vi "Write Post Office Addresses.vi"(8 "error in (no error)":errorcluster, 10 "Post Office Addresses":string[](array[string]), 11 "Post in":refnum<class "Post.lvclass">) -> (0 "error out":errorcluster, 3 "Post out":refnum<class "Post.lvclass">)   [LabVIEW 2019, in "Post.lvclass"]
uses:
  Post.lvclass
  Post.lvclass/Post.ctl
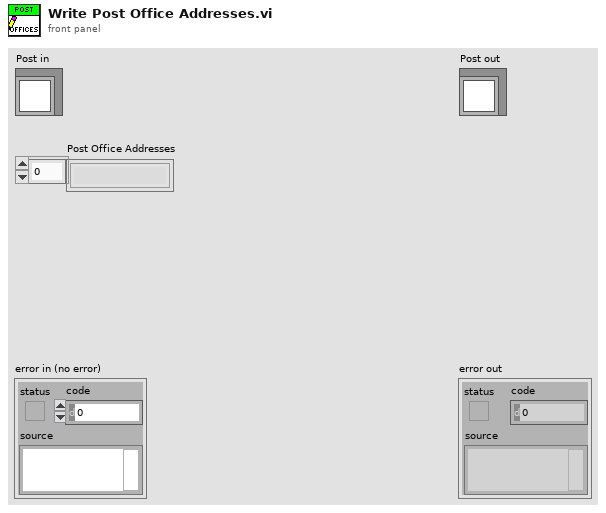
[diagram p1: front panel]
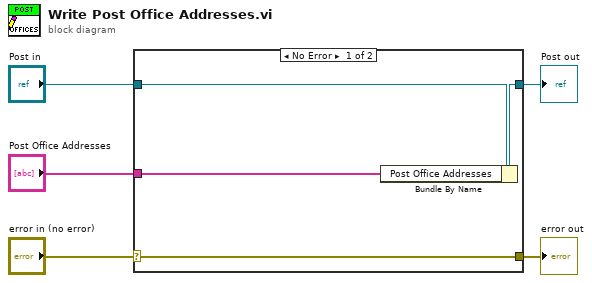
[diagram p0: block diagram]
diagram:
  n1 = case shown="No Error" "error in (no error)" {
    selector: "error in (no error)" -> [w9 w10]
    tunnel: [w9 w10] -> w4
    tunnel: [w7 w11] -> w2
    tunnel: "Post in" -> [w8 w11]
    tunnel: "Post Office Addresses" -> [w6 _]
    frame No Error {
      n2 = Bundle By Name(cluster=w8, "Post Office Addresses"=w6) -> (w7:refnum<class "Post.lvclass">)
    }
    frame Error {
    }
  }
  "error out" <- w4
  "Post out" <- w2
